vi "Compute Distance (V+H).vi"(10 "point 2":cluster{"x":i64, "y":i64}, 11 "point 1":cluster{"x":i64, "y":i64}) -> (3 "distance":u64)   [LabVIEW 2022 SP3]
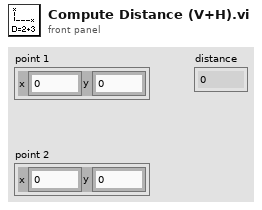
[diagram p1: front panel]
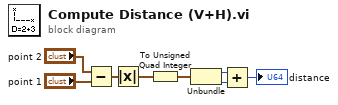
[diagram p0: block diagram]
diagram:
  n1 = Subtract(x="point 2", y="point 1") -> (x-y=w4:cluster{"x":i64, "y":i64})
  n2 = Absolute Value(x=w4) -> (abs(x)=w5:cluster{"x":i64, "y":i64})
  n3 = To Unsigned Quad Integer(1:w5) -> (0:w1:cluster{"x":u64, "y":u64})
  n4 = Unbundle(w1) -> ("x"=w6:u64, "y"=w7:u64)
  n5 = Add(x=w6, y=w7) -> (x+y=→"distance":u64)
